vi "Read.vi"(8 "error in (no error)":errorcluster, 10 "byte count":u32, 11 "Simulated Serial in":refnum<class "Simulated Serial.lvclass">) -> (0 "error out":errorcluster, 2 "read buffer":string, 3 "Simulated Serial out":refnum<class "Simulated Serial.lvclass">)   [LabVIEW 2020, in "Simulated Serial.lvclass"]
uses:
  Simulated Serial.lvclass
  Simulated Serial.lvclass/Simulated Serial.ctl
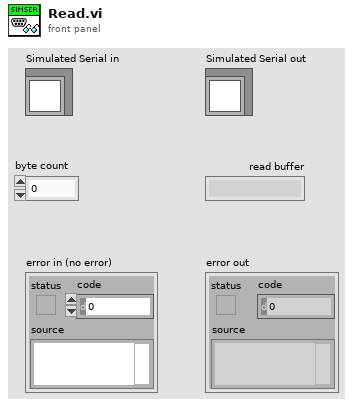
[diagram p1: front panel]
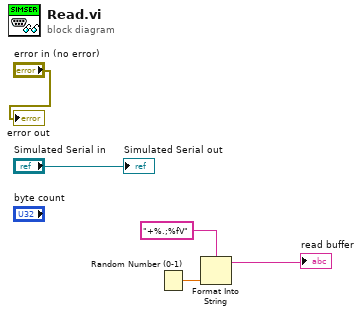
[diagram p0: block diagram]
diagram:
  n1 = Random Number (0-1)() -> (number: 0 to 1=w3:dbl)
  n2 = Format Into String(format string="+%.;%fV", w3) -> (resulting string=→"read buffer":string)  [unwired: 2 in, 1 out]
  "error out" <- "error in (no error)"
  "Simulated Serial out" <- "Simulated Serial in"
